vi "test_ccd_convertWavelengthToRamanShift.vi"(8 "error in (no error)":errorcluster) -> (0 "error out":errorcluster)   [LabVIEW 2023, in "horiba.test.lvlib"]
uses:
  horiba.test.lvlib
  <vilib>/addons/_JKI Toolkits/Caraya/classes/Assert/Assert Almost Equal_Float.vi
  <vilib>/addons/_JKI Toolkits/Caraya/classes/Test/Test.lvclass
  <vilib>/addons/_JKI Toolkits/Caraya/classes/Assert/Assert.lvclass
  Classes/CCD/CCD.lvclass
panel:
  out "Array":dbl[](array[numeric])
  # "Connector Pane"
  # "Locals"
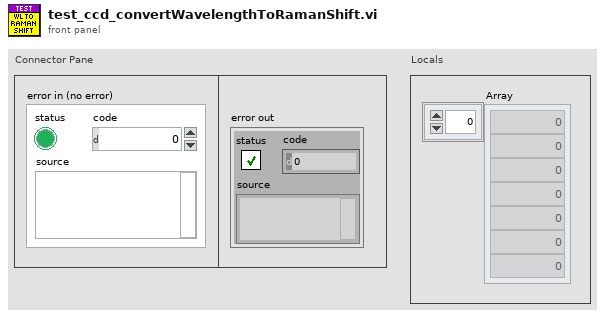
[diagram p1: front panel]
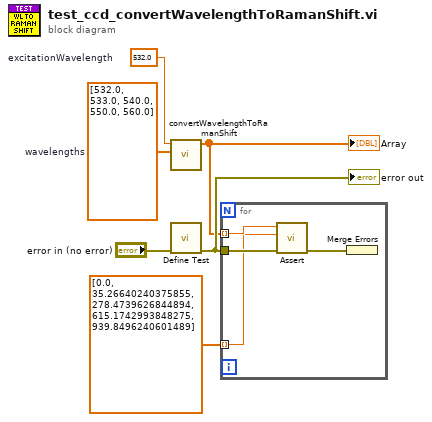
[diagram p0: block diagram]
diagram:
  w4 = 532.0  # excitationWavelength
  w3 = dbl[] [532.0, 533.0, 540.0, 550.0, 560.0]  # wavelengths
  n1 = call "convertWavelengthToRamanShift.vi"("wavelengths"=w3, "excitationWavelength"=w4) -> ("Array"=w2:dbl[])  [unwired: 9 in]
  "Array" <- w2
  n2 = call <vilib>:"Define Test.vi"("error in (no error)"="error in (no error)") -> ("error out"=w6:errorcluster)  [unwired: 9 in, 1 out]
  "error out" <- w6
  n3 = for {
    tunnel: w6 -> [w9]
    tunnel: w2 -> [w8] mode=indexing
    tunnel: dbl[] [0.0, 35.26640240375855, 278.4739626844894, 615.1742993848275, 939.8496240601489] ("ramanShifts") -> [w7] mode=indexing
    n4 = call-poly <vilib>:"Assert.vi"("error in (no error)"=w9, "Y"=w7, "X"=w8) -> ("error out"=w10:errorcluster)  [unwired: 7 in, 1 out]
    n5 = Merge Errors(w10) -> ()  [unwired: 1 out]
  }
